vi "FPGA.vi"() -> ()   [LabVIEW 2013]
uses:
  PMUmeasurements.ctl
  ToFPGA.ctl
  <vilib>/rvi/Emulation/niFpgaSctlEmulationGetInTimedLoop.vi
  <vilib>/rvi/Emulation/niFpgaEmulationReportErrorSimple.vi
  <vilib>/rvi/Emulation/niFpgaGetClockAttributes.vi
  <vilib>/rvi/eio/common/nirviEmuTemplateMethod_errors.vi
  <vilib>/rvi/Emulation/niFpgaCriticalErrorInLSC.vi
  <vilib>/eio/EIONode/EIONode.xnode
panel:
  in  "FGPA Loop Timer":u8 caption="Count(uSec)"
  out "Loop period monitoring":u8
  out "The output signals":T1
  out "FPGA Error Out":errorcluster
  in  "PMU measurments":T2
  in  "stop":bool
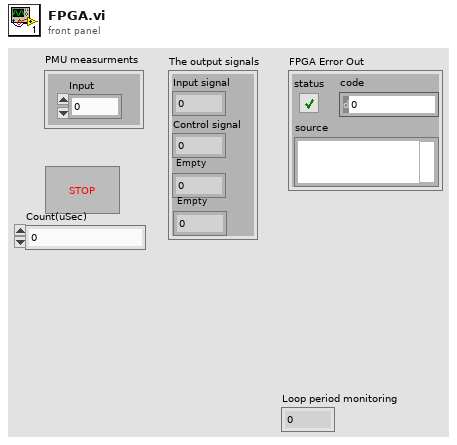
[diagram p1: front panel]
types:
  T1 = typedef "ToFPGA.ctl" = cluster{"Input signal":sgl, "Control signal":sgl, " Empty":sgl, " Empty":sgl}
  T2 = typedef "PMUmeasurements.ctl" = cluster{"Input":sgl}
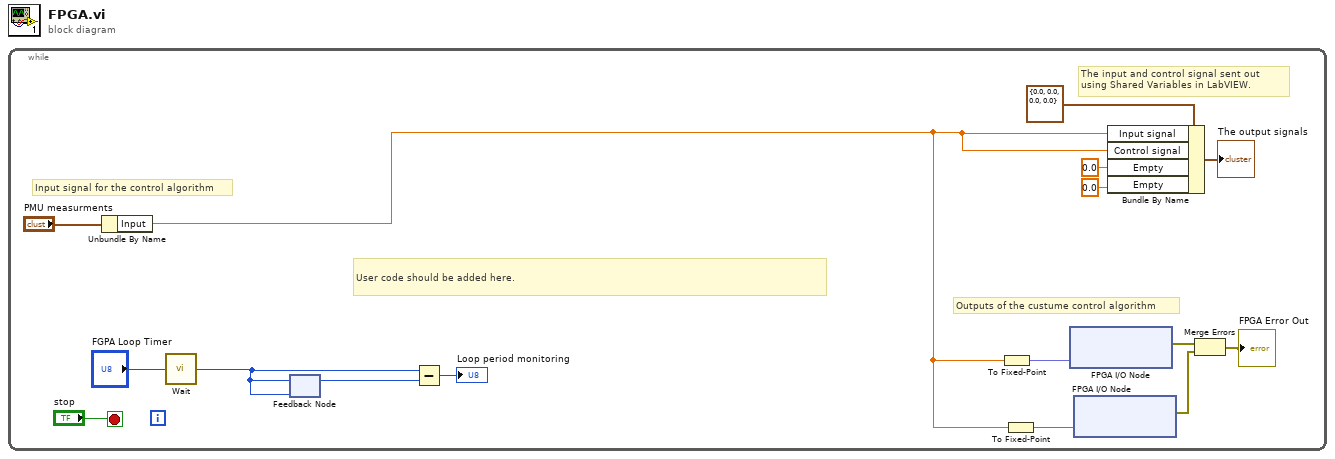
[diagram p0: block diagram]
diagram:
  n1 = while {
    stop <- "stop" stop-if-true
    # "Outputs of the custume control algorithm"
    # "User code should be added here."
    # "The input and control signal sent out using Shared Variables in LabVIEW."
    # "Input signal for the control algorithm"
    n2 = Unbundle By Name("PMU measurments") -> ("Input"=w7:sgl)
    n3 = call "Wait"("Count(uSec)"="FGPA Loop Timer") -> ("Tick Count(uSec)"=w2:u8)
    n4 = feedback #1(w2) -> (w3:u8)
    n5 = feedback-in #1(w2) -> ()
    n6 = Subtract(x=w2, y=w3) -> (x-y=→"Loop period monitoring":u8)
    n7 = To Fixed-Point(number=w7) -> (fixed-point=w8:fxp<+/-,20,5>)  [unwired: 1 in]
    n8 = To Fixed-Point(number=w7) -> (fixed-point=w13:fxp<+/-,20,5>)  [unwired: 1 in]
    n9 = xnode "FPGA I/O Node"("Mod1/AO1"=w8) -> ("error out"=w12:errorcluster)  [unwired: 2 in, 1 out]
    n10 = xnode "FPGA I/O Node"("Mod1/AO0"=w13) -> ("error out"=w11:errorcluster)  [unwired: 2 in, 1 out]
    n11 = Bundle By Name(cluster=T1 {"Input signal"=0.0, "Control signal"=0.0, " Empty"=0.0, " Empty"=0.0}, "Input signal"=w7, "Control signal"=w7, "Empty"=sgl 0.0, "Empty"=sgl 0.0) -> (→"The output signals":T1)
    n12 = Merge Errors(w12, w11) -> (→"FPGA Error Out":errorcluster)
  }
